vi "Harv_2_9.vi"(6 "Harvest":bool, 7 "Fire":bool, 8 "FireBallSen":bool, 9 "BallAcquired":bool, 10 "HarvPot":dbl, 11 "HarvSetpoints":dbl[](array[numeric])) -> (0 "HarvCleared":bool, 2 "HarvRoller":dbl, 3 "HarvPower":dbl)   [LabVIEW 2013]
panel:
  in  "MotorScale":dbl=1.5
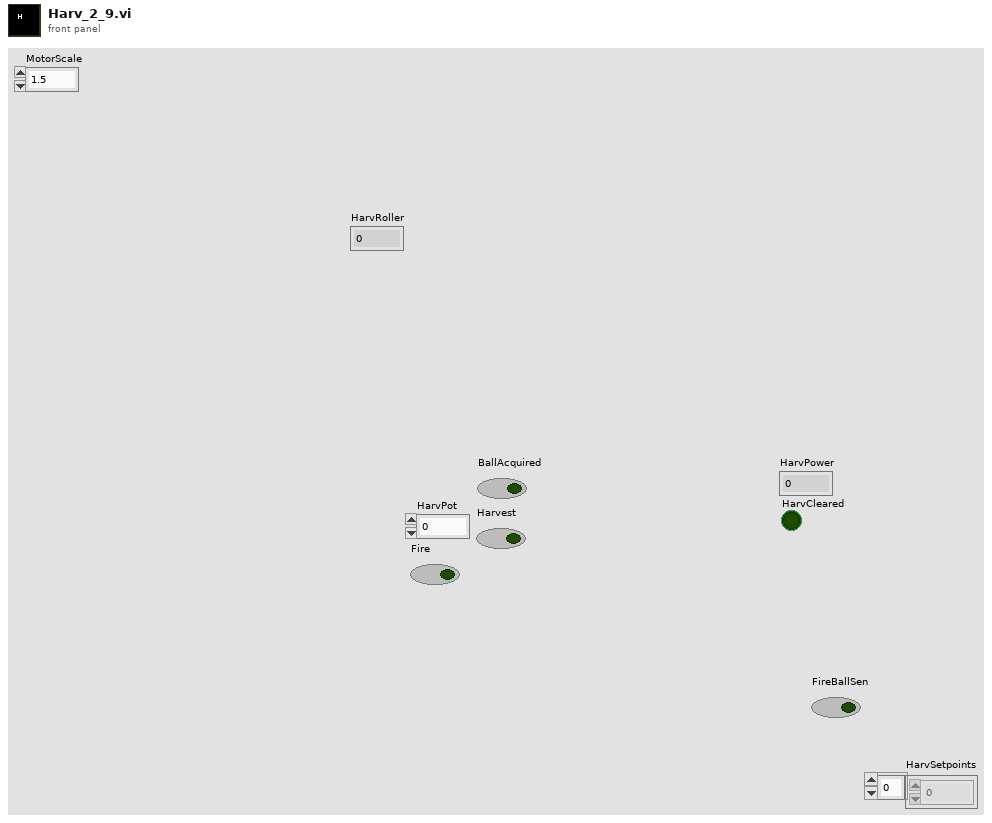
[diagram p1: front panel]
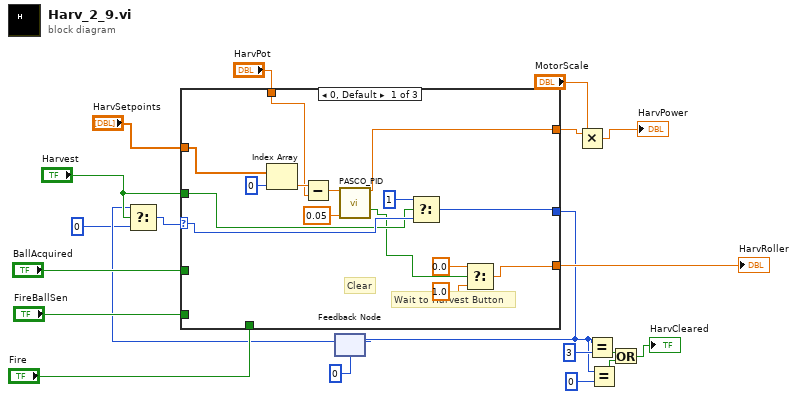
[diagram p0: block diagram]
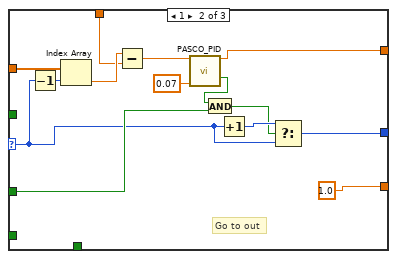
[diagram p2: hidden frame]
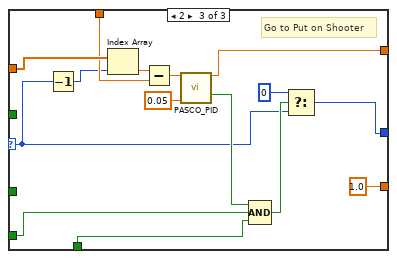
[diagram p3: hidden frame]
diagram:
  n1 = feedback #1(0 ("Numeric")) -> (w5:i32)
  n2 = Select(t=w5, s="Harvest", f=0) -> (s? t:f=w7:i32)
  n3 = case shown="0, Default" w7 {
    selector: w7 -> [w30 w37 w52]
    tunnel: "HarvSetpoints" -> [w29 w49 w63]
    tunnel: "HarvPot" -> [w28 w47 w61]
    tunnel: [w27 w45 w59] -> w3
    tunnel: [w26 w43 w58] -> w9
    tunnel: [w25 1.0 1.0] -> w18
    tunnel: "BallAcquired" -> [_ w39 _]
    tunnel: "FireBallSen" -> [_ _ w55]
    tunnel: "Fire" -> [_ _ w54]
    tunnel: "Harvest" -> [w24 _ _]
    frame 0, Default {
      # "Clear"
      # "Wait to Harvest Button"
      n4 = Index Array(array=w29, index=0) -> (element=w31:dbl)
      n5 = Subtract(x=w31, y=w28) -> (x-y=w32:dbl)
      n6 = call "PASCO_PID.vi"("Delta"=w32, "Deadband"=0.05) -> ("Output"=w27:dbl, "IsThere"=w23:bool)  [unwired: 12 in]
      n7 = Select(t=1, s=w24, f=w30) -> (s? t:f=w26:i32)
      n8 = Select(t=0.0, s=w23, f=1.0) -> (s? t:f=w25:dbl)
    }
    frame 1 {
      # "Go to out"
      n9 = Decrement(x=w37) -> (x-1=w38:i32)
      n10 = Index Array(array=w49, index=w38) -> (element=w48:dbl)
      n11 = Subtract(x=w48, y=w47) -> (x-y=w46:dbl)
      n12 = call "PASCO_PID.vi"("Delta"=w46, "Deadband"=0.07) -> ("Output"=w45:dbl, "IsThere"=w41:bool)  [unwired: 12 in]
      n13 = And(x=w41, y=w39) -> (x .and. y?=w40:bool)
      n14 = Increment(x=w37) -> (x+1=w44:i32)
      n15 = Select(t=w44, s=w40, f=w37) -> (s? t:f=w43:i32)
    }
    frame 2 {
      # "Go to Put on Shooter"
      n16 = Decrement(x=w52) -> (x-1=w53:i32)
      n17 = Index Array(array=w63, index=w53) -> (element=w62:dbl)
      n18 = Subtract(x=w62, y=w61) -> (x-y=w60:dbl)
      n19 = call "PASCO_PID.vi"("Delta"=w60, "Deadband"=0.05) -> ("Output"=w59:dbl, "IsThere"=w56:bool)  [unwired: 12 in]
      n20 = Compound Arithmetic op=AND(w56, w55, w54) -> (w57:bool)
      n21 = Select(t=0, s=w57, f=w52) -> (s? t:f=w58:i32)
    }
  }
  "HarvRoller" <- w18
  n22 = feedback-in #1(w9) -> ()
  n23 = Multiply(x=w3, y="MotorScale") -> (x*y=→"HarvPower":dbl)
  n24 = Equal?(x=w9, y=3) -> (x = y?=w11:bool)
  n25 = Equal?(x=w9, y=0) -> (x = y?=w12:bool)
  n26 = Or(x=w11, y=w12) -> (x .or. y?=→"HarvCleared":bool)
